vi "SetParam.vi"(8 "error in (no error)":errorcluster caption="entrée d'erreur (pas d'erreur)", 10 "label_ranking_average_precision_score":cluster{"sample_weight":dbl[]}, 11 "Label_Ranking_Average_PS in":refnum<class "Label_Ranking_Average_PS.lvclass">) -> (0 "error out":errorcluster caption="sortie d'erreur", 3 "Label_Ranking_Average_PS out":refnum<class "Label_Ranking_Average_PS.lvclass">)   [LabVIEW 2020, in "Label_Ranking_Average_PS.lvclass"]
doc: "Set parameters"
uses:
  Label_Ranking_Average_PS.lvclass
  Label_Ranking_Average_PS.lvclass/Label_Ranking_Average_PS.ctl
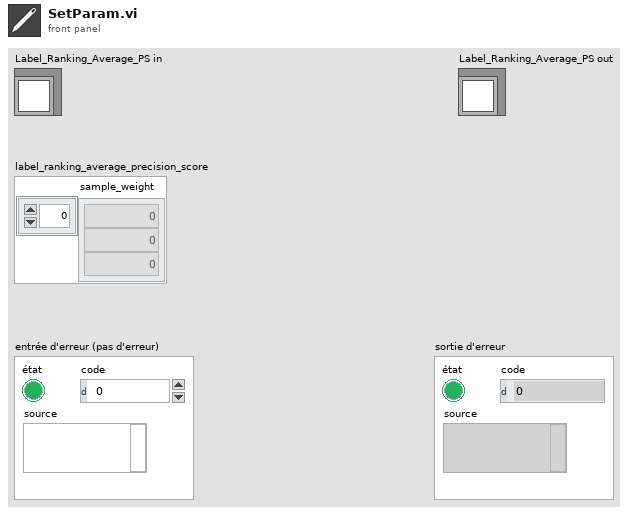
[diagram p1: front panel]
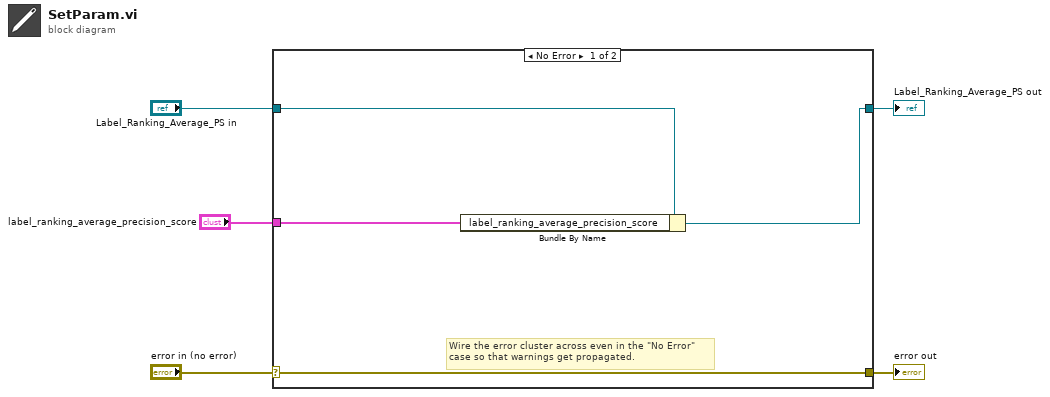
[diagram p0: block diagram]
diagram:
  n1 = case shown="No Error" "error in (no error)" {
    selector: "error in (no error)" -> [w9 w11]
    tunnel: [w9 w11] -> w4
    tunnel: [w6 w10] -> w2
    tunnel: "Label_Ranking_Average_PS in" -> [w7 w10]
    tunnel: "label_ranking_average_precision_score" -> [w8 _]
    frame No Error {
      # "Wire the error cluster across even in the \"No Error\"\ncase so that warnings get propagated."
      n2 = Bundle By Name(cluster=w7, "label_ranking_average_precision_score"=w8) -> (w6:refnum<class "Label_Ranking_Average_PS.lvclass">)
    }
    frame Error {
    }
  }
  "error out" <- w4
  "Label_Ranking_Average_PS out" <- w2
